vi "format unc and dof by value.vi"(9 "vector dof":dbl[](array[numeric]) caption="DoF", 10 "vector unc":dbl[](array[numeric]) caption="Uncertainty", 11 "vector value":dbl[](array[numeric]) caption="Value") -> (1 "vector dof out":dbl[](array[numeric]), 2 "vector unc out":dbl[](array[numeric]), 3 "vector value out":dbl[](array[numeric]) caption="Value")   [LabVIEW 2013]
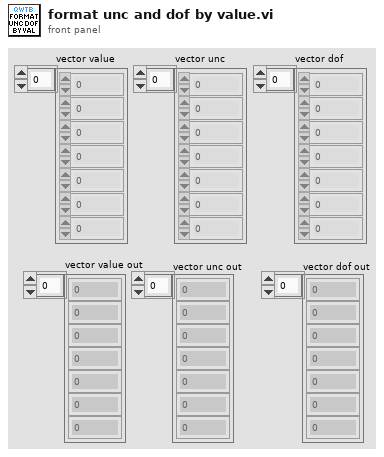
[diagram p1: front panel]
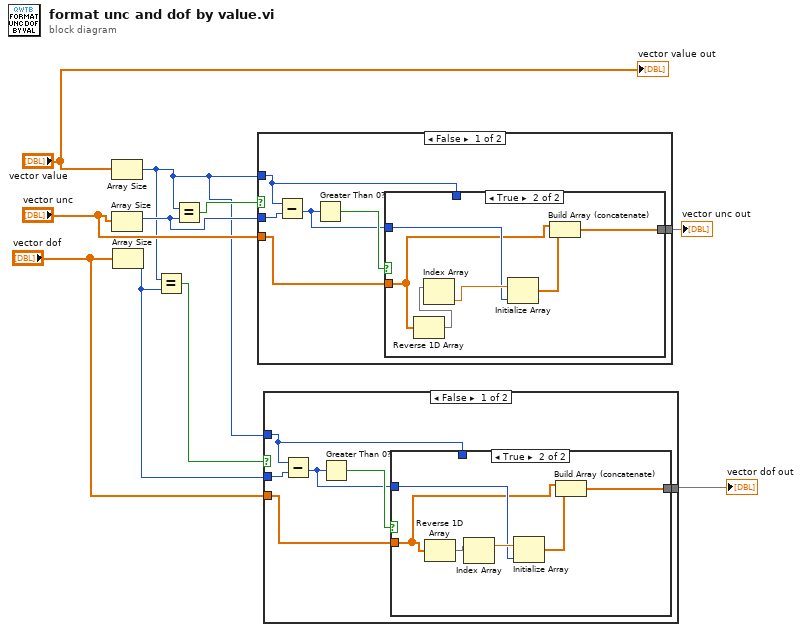
[diagram p0: block diagram]
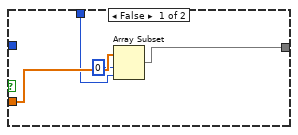
[diagram p2: hidden frame]
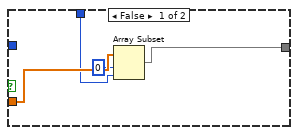
[diagram p4: hidden frame]
diagram:
  n1 = Array Size(array="vector value") -> (size(s)=w3:i32)
  n2 = Array Size(array="vector unc") -> (size(s)=w7:i32)
  n3 = Array Size(array="vector dof") -> (size(s)=w4:i32)
  n4 = Equal?(x=w3, y=w4) -> (x = y?=w2:bool)
  n5 = Equal?(x=w3, y=w7) -> (x = y?=w9:bool)
  n6 = case shown="False" w9 {
    tunnel: [w12 w27] -> w6
    tunnel: "vector unc" -> [w16 w27]
    tunnel: w3 -> [w11 _]
    tunnel: w7 -> [w15 _]
    frame False {
      n7 = Subtract(x=w11, y=w15) -> (x-y=w13:i32)
      n8 = Greater Than 0?(x=w13) -> (x > 0?=w14:bool)
      n9 = case shown="True" w14 {
        tunnel: w16 -> [w20 w22]
        tunnel: w13 -> [_ w25]
        tunnel: [w17 w23] -> w12
        tunnel: w11 -> [w18 _]
        frame False {
          n10 = Array Subset(array=w20, index=0, length=w18) -> (w17:dbl[])
        }
        frame True {
          n11 = Reverse 1D Array(array=w22) -> (reversed array=w21:dbl[])
          n12 = Index Array(array=w21) -> (element=w26:dbl)  [unwired: 1 in]
          n13 = Initialize Array(w26, w25) -> (w24:dbl[])
          n14 = Build Array (concatenate)(w22, w24) -> (w23:dbl[])
        }
      }
    }
    frame True {
    }
  }
  "vector unc out" <- w6
  n15 = case shown="False" w2 {
    tunnel: [w29 w44] -> w1
    tunnel: "vector dof" -> [w33 w44]
    tunnel: w3 -> [w28 _]
    tunnel: w4 -> [w32 _]
    frame False {
      n16 = Subtract(x=w28, y=w32) -> (x-y=w30:i32)
      n17 = Greater Than 0?(x=w30) -> (x > 0?=w31:bool)
      n18 = case shown="True" w31 {
        tunnel: w33 -> [w37 w39]
        tunnel: w30 -> [_ w42]
        tunnel: [w34 w40] -> w29
        tunnel: w28 -> [w35 _]
        frame False {
          n19 = Array Subset(array=w37, index=0, length=w35) -> (w34:dbl[])
        }
        frame True {
          n20 = Reverse 1D Array(array=w39) -> (reversed array=w38:dbl[])
          n21 = Index Array(array=w38) -> (element=w43:dbl)  [unwired: 1 in]
          n22 = Initialize Array(w43, w42) -> (w41:dbl[])
          n23 = Build Array (concatenate)(w39, w41) -> (w40:dbl[])
        }
      }
    }
    frame True {
    }
  }
  "vector dof out" <- w1
  "vector value out" <- "vector value"
